vi "v5.4.vi"() -> ()   [LabVIEW 2018]
uses:
  <vilib>/DAQmx/read.llb/DAQmx Read (Analog 1D DBL NChan 1Samp).vi
  <extravilib>/ChannelInstances/Lossy Stream-c(a[.](c(dbl,dbl,dbl,dbl)),stamp,a[.](dbl),c(dbl,dbl,dbl,dbl,dbl,dbl,dbl))/Read With Abort.vi
  <extravilib>/ChannelInstances/High Speed Stream-c(a[.](c(dbl,dbl,dbl,dbl)),stamp,a[.](dbl),c(dbl,dbl,dbl,dbl,dbl,dbl,dbl))/_Read For Replicate.vi
  <extravilib>/ChannelInstances/Lossy Stream-c(a[.](c(dbl,dbl,dbl,dbl)),stamp,a[.](dbl),c(dbl,dbl,dbl,dbl,dbl,dbl,dbl))/Write With Abort.vi
  <extravilib>/ChannelInstances/Lossy Stream-c(a[.](c(dbl,dbl,dbl,dbl)),stamp,a[.](dbl),c(dbl,dbl,dbl,dbl,dbl,dbl,dbl))/EndpointRead.vi
  <extravilib>/ChannelInstances/Lossy Stream-c(a[.](c(dbl,dbl,dbl,dbl)),stamp,a[.](dbl),c(dbl,dbl,dbl,dbl,dbl,dbl,dbl))/Endpoint.vi
  <extravilib>/ChannelInstances/Lossy Stream-c(a[.](c(dbl,dbl,dbl,dbl)),stamp,a[.](dbl),c(dbl,dbl,dbl,dbl,dbl,dbl,dbl))/Instantiate.vi
  <extravilib>/ChannelInstances/Lossy Stream-c(a[.](c(dbl,dbl,dbl,dbl)),stamp,a[.](dbl),c(dbl,dbl,dbl,dbl,dbl,dbl,dbl))/)Channel.vi
  <resource>/ChannelSupport/_ChannelSupport/WaitIfNeeded.vi
  <extravilib>/ChannelInstances/High Speed Stream-c(a[.](c(dbl,dbl,dbl,dbl)),stamp,a[.](dbl),c(dbl,dbl,dbl,dbl,dbl,dbl,dbl))/Instantiate.vi
  <extravilib>/ChannelInstances/High Speed Stream-c(a[.](c(dbl,dbl,dbl,dbl)),stamp,a[.](dbl),c(dbl,dbl,dbl,dbl,dbl,dbl,dbl))/)Channel.vi
  <extravilib>/ChannelInstances/High Speed Stream-c(a[.](c(dbl,dbl,dbl,dbl)),stamp,a[.](dbl),c(dbl,dbl,dbl,dbl,dbl,dbl,dbl))/Abort Signal/Init Signal.vi
  <vilib>/Utility/file.llb/Write Delimited Spreadsheet (string).vi
  <vilib>/DAQmx/create/channels.llb/DAQmx Create Channel (AI-Temperature-Thermocouple).vi
  <vilib>/DAQmx/configure/timing.llb/DAQmx Timing (Sample Clock).vi
  <vilib>/DAQmx/miscellaneous.llb/DAQmx Fill In Error Info.vi
  <extravilib>/ChannelInstances/High Speed Stream-c(a[.](c(dbl,dbl,dbl,dbl)),stamp,a[.](dbl),c(dbl,dbl,dbl,dbl,dbl,dbl,dbl)).lvlib
  <resource>/objmgr/daqmx.rc
  <extravilib>/ChannelInstances/Lossy Stream-c(a[.](c(dbl,dbl,dbl,dbl)),stamp,a[.](dbl),c(dbl,dbl,dbl,dbl,dbl,dbl,dbl)).lvlib
panel:
  in  "Rig Temperature Tab Box":enum32{"Rig Temps Live", "Alarm Thresholds"}(tab)
  out "Rig Temperatures":T1
  in  "Rig Alarm Thresholds":T1
  out "DAQ Current Time":timestamp format="%<%X>T"
  in  "UI Refresh Rate (Hz)":u32=1 min=1 max=500 step=1
  out "Line Pressures":T2(graph)
  in  "Boondoggle":dbl(slide) scale=0.0..10.0
  out "Line Temperatures":T2(graph)
  out "Stoichiometric AFR [g/s]":dbl
  in  "stop":bool
  in  "Species List":string[][](table)=[["Custom", "9999999999"], ["Methanol", "6.47"], ["Butanol", "11.2"], ["Diesel", "14.5"], ["Gasoline", "14.7"], ["Propane", "15.67"], ["Methane", "13.19"], ["Hydrogen", "34.3"], ["Ammonia", "6.0466"], ["Pentane", "15.32"], ["Butane", "14.98"], ["Hexane", "15.24"], ["Ethanol", "9"], ["Empty (Not Used)", "0"]]
  in  "Lines Tab Control\n(Don't delete)":enum32{"Live Data", "AFR Info", "Setup Lines"}(tab)
  out "Flowrate Data":T3(array[cluster])
  out "AFR Display":T4(array[cluster])
  in  "Line Setup":T5(array[cluster])
  out "Actual Sample Rate":dbl
  out "Export Timestamp":timestamp format="%<%H:%M:%S>T"
  out "UI Timestamp":timestamp format="%<%X\n%x>T"
  in  "file path (dialog if empty)":path
  out "Export Loop Status":T6(ring)
  in  "Start Recording?":bool
  in  "Stop Recording?":bool
  out "Aquisition\nLoop Status":T7(ring)
  in  "OK Button":bool
  in  "DAQ Properties":cluster{"Sample Rate [Hz]":dbl}={"Sample Rate [Hz]"=1.0} {"Sample Rate [Hz]" min=1.0 max=500.0 step=1.0}
  # "Rig Temperatures [ °C]"
  # "Rig Alarm Thresholds [ °C]"
  # "Live \n Live Line Data"
  # "Air-to-Fuel Ratios for each Line"
  # "Line Setup"
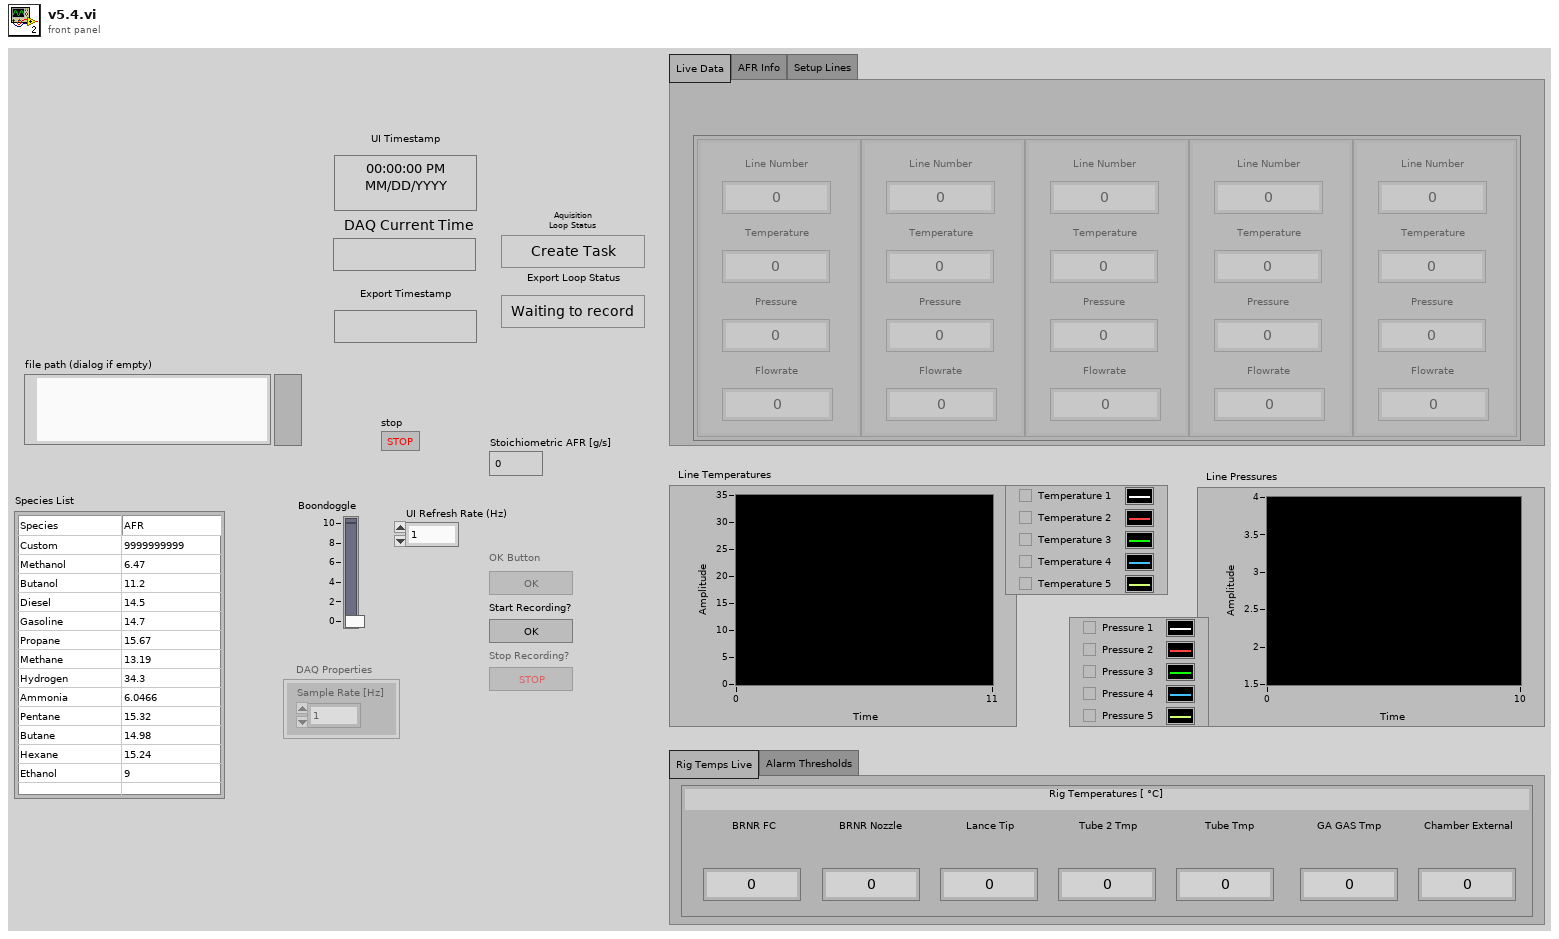
[diagram p1: front panel]
types:
  T1 = cluster{"BRNR FC":dbl, "BRNR Nozzle":dbl, "Lance Tip":dbl, "Tube 2 Tmp":dbl, "Tube Tmp":dbl, "GA GAS Tmp":dbl, "Chamber External":dbl}
  T2 = cluster{"[0]":dbl, "[1]":dbl, "[2]":dbl, "[3]":dbl, "[4]":dbl}
  T3 = cluster{"Line Number":dbl, "Temperature":dbl, "Pressure":dbl, "Flowrate":dbl}[]
  T4 = cluster{"Line Number":i32, "AFR":dbl, "Species":enum16{"Empty (Not used)", "Custom", "Methanol", "Ethanol", "Butanol", "Diesel", "Gasoline", "Propane", "Methane", "Hydrogen", "Pentane", "Butane", "Hexane"}}[]
  T5 = cluster{"Custom AFR":dbl, "Species":enum16{"Empty (Not used)", "Custom", "Methanol", "Ethanol", "Butanol", "Diesel", "Gasoline", "Propane", "Methane", "Hydrogen", "Pentane", "Butane", "Hexane"}}[]
  T6 = enum16{"Waiting to record", "Creating Spreadsheet", "Recording", "Finished Recording"}
  T7 = enum16{"Create Task", "Change Settings", "Check Settings", "Read Data", "End Task"}
  T8 = enum8{"Enabled", "Disabled", "Disabled and Grayed Out"}
  T9 = cluster{"Line":i32, "AFR":dbl, "Species":enum16{"Empty (Not used)", "Custom", "Methanol", "Ethanol", "Butanol", "Diesel", "Gasoline", "Propane", "Methane", "Hydrogen", "Pentane", "Butane", "Hexane"}}
  T10 = enum16{"Empty (Not used)", "Custom", "Methanol", "Ethanol", "Butanol", "Diesel", "Gasoline", "Propane", "Methane", "Hydrogen", "Pentane", "Butane", "Hexane"}
  T11 = cluster{"Flowrate Data":cluster{"Line Number":dbl, "Temperature":dbl, "Pressure":dbl, "Flowrate":dbl}[], "Current Time":timestamp, "DAQmx Data":dbl[], "Rig Temperatures":cluster{"BRNR FC":dbl, "BRNR Nozzle":dbl, "Lance Tip":dbl, "Tube 2 Tmp":dbl, "Tube Tmp":dbl, "GA GAS Tmp":dbl, "Chamber External Temp":dbl}}
  T12 = cluster{"BRNR FC":dbl, "BRNR Nozzle":dbl, "Lance Tip":dbl, "Tube 2 Tmp":dbl, "Tube Tmp":dbl, "GA GAS Tmp":dbl, "Chamber External Temp":dbl}
  T13 = typedef "High Speed Stream-c(a[.](c(dbl,dbl,dbl,dbl)),stamp,a[.](dbl),c(dbl,dbl,dbl,dbl,dbl,dbl,dbl)).lvlib/)Channel.ctl" = refnum<queue>
  T14 = typedef "Lossy Stream-c(a[.](c(dbl,dbl,dbl,dbl)),stamp,a[.](dbl),c(dbl,dbl,dbl,dbl,dbl,dbl,dbl)).lvlib/)Channel.ctl" = refnum<queue>
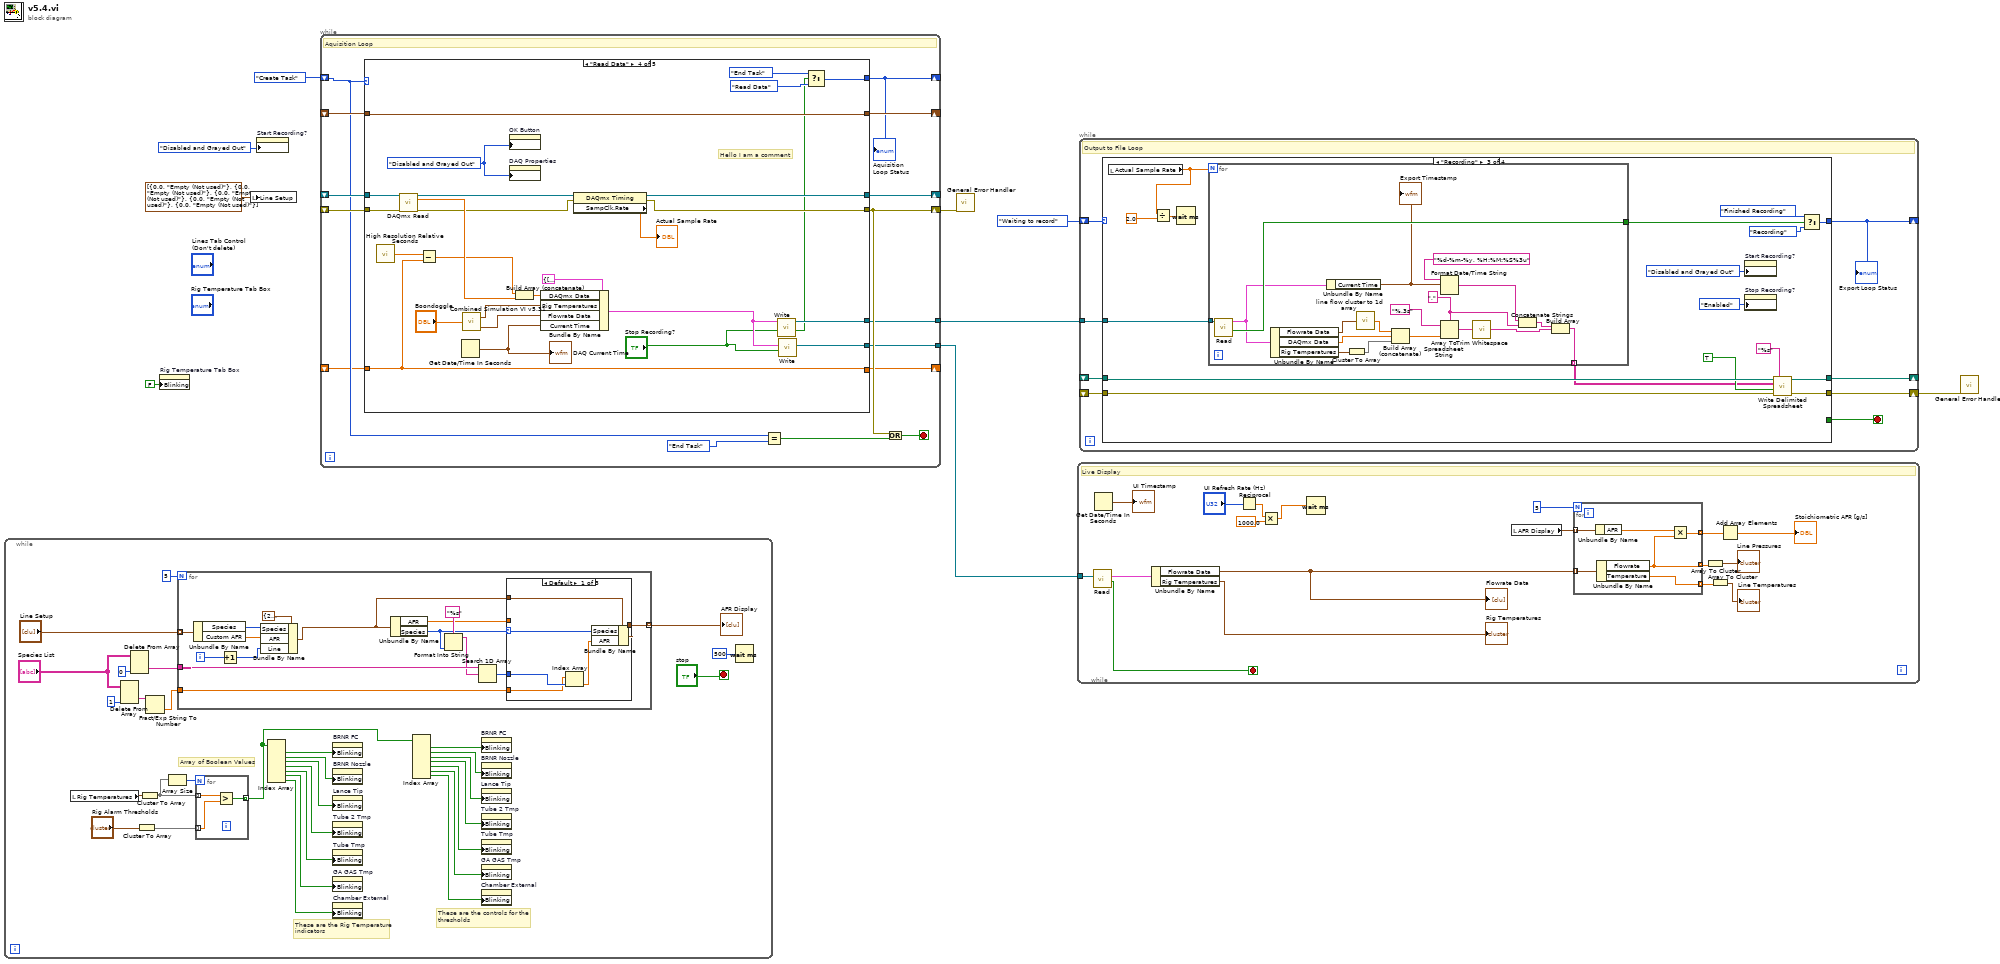
[diagram p0: block diagram]
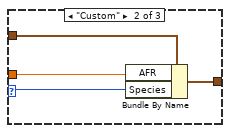
[diagram p2: hidden frame]
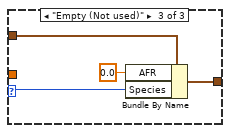
[diagram p3: hidden frame]
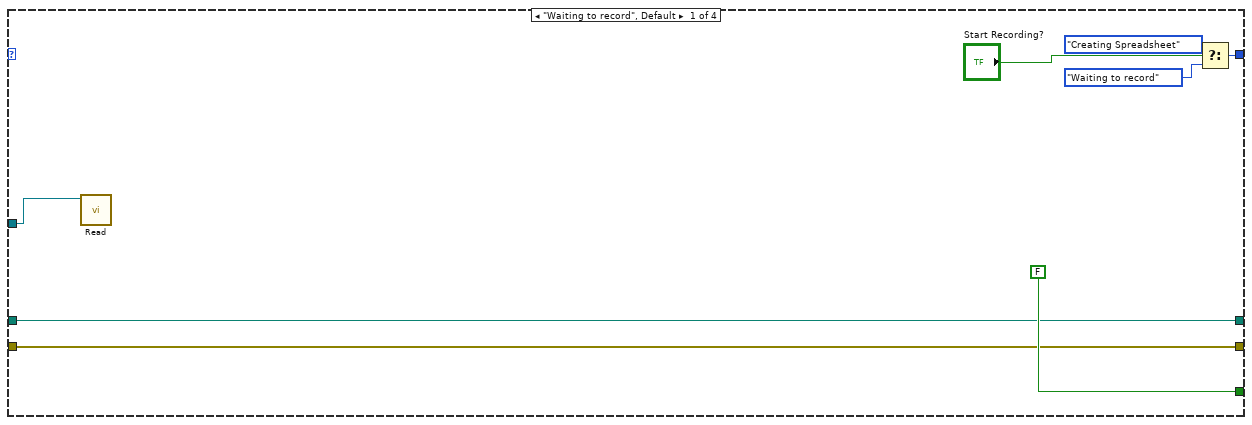
[diagram p4: hidden frame]
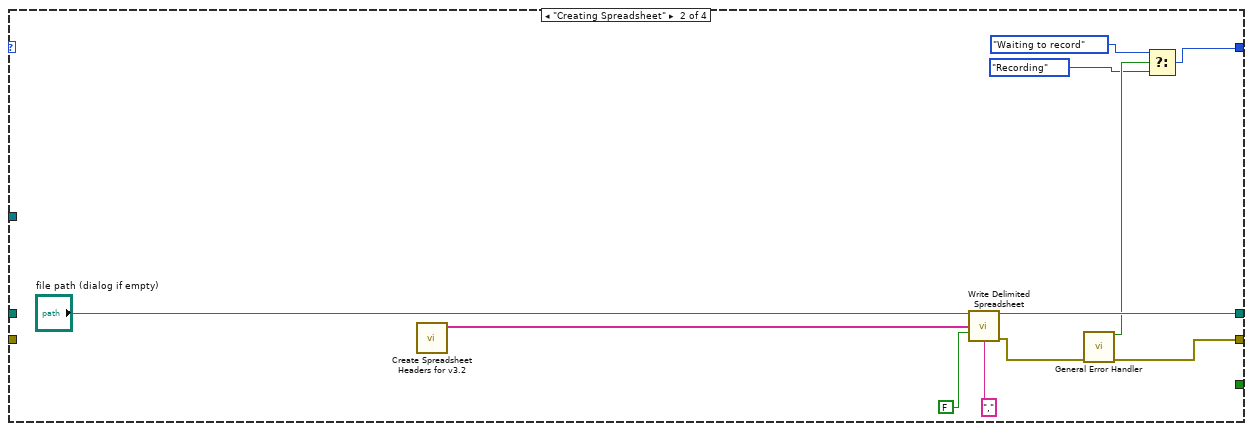
[diagram p5: hidden frame]
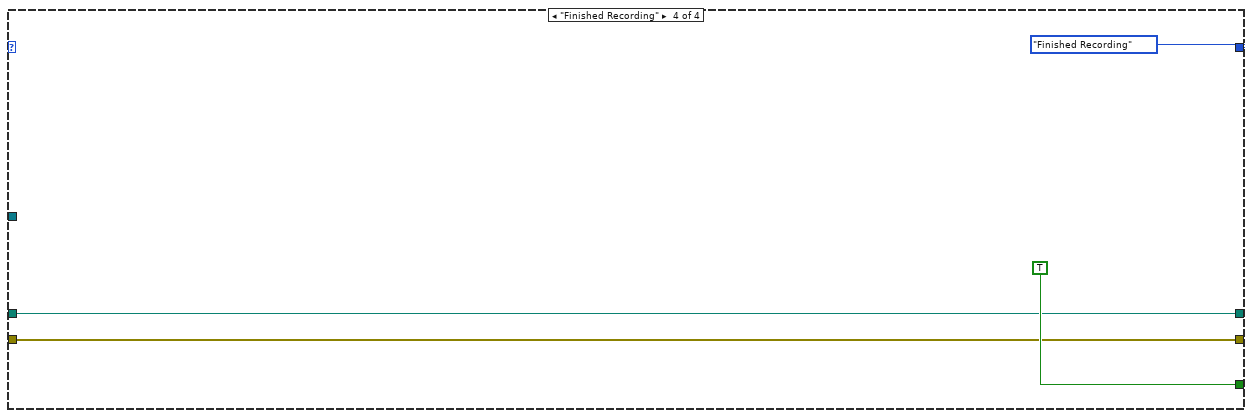
[diagram p6: hidden frame]
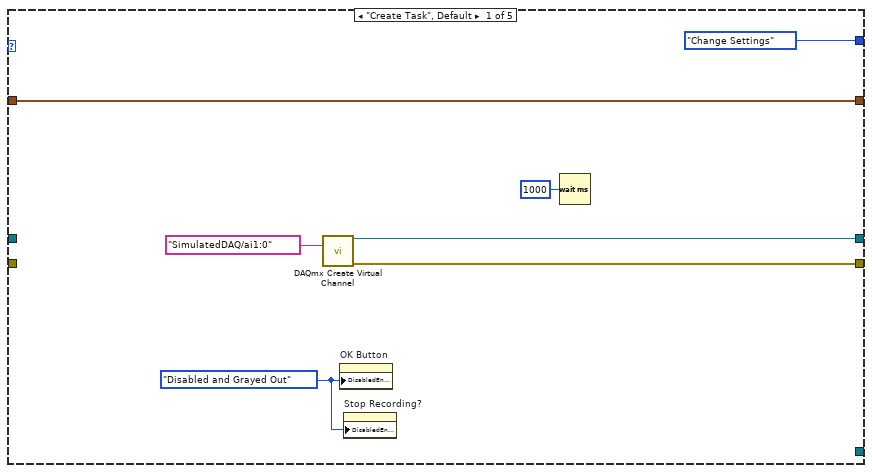
[diagram p7: hidden frame]
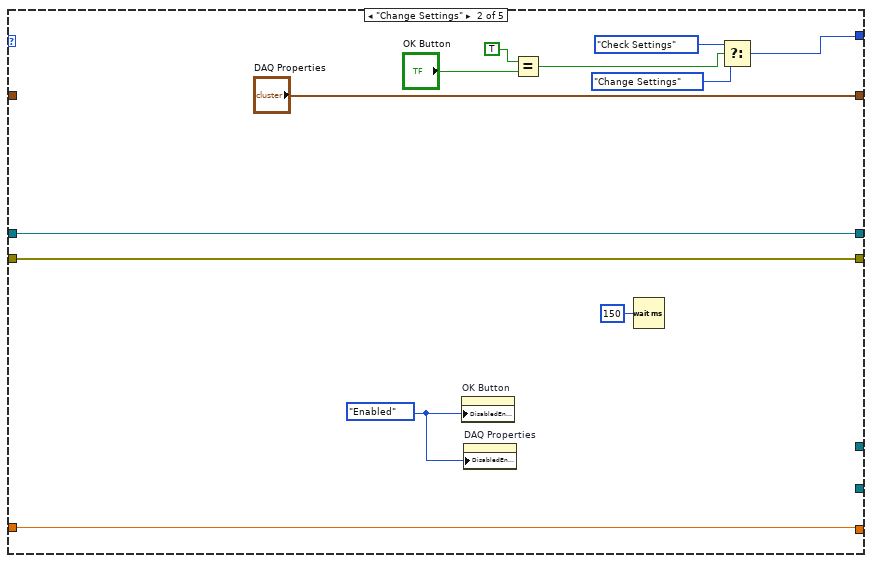
[diagram p8: hidden frame]
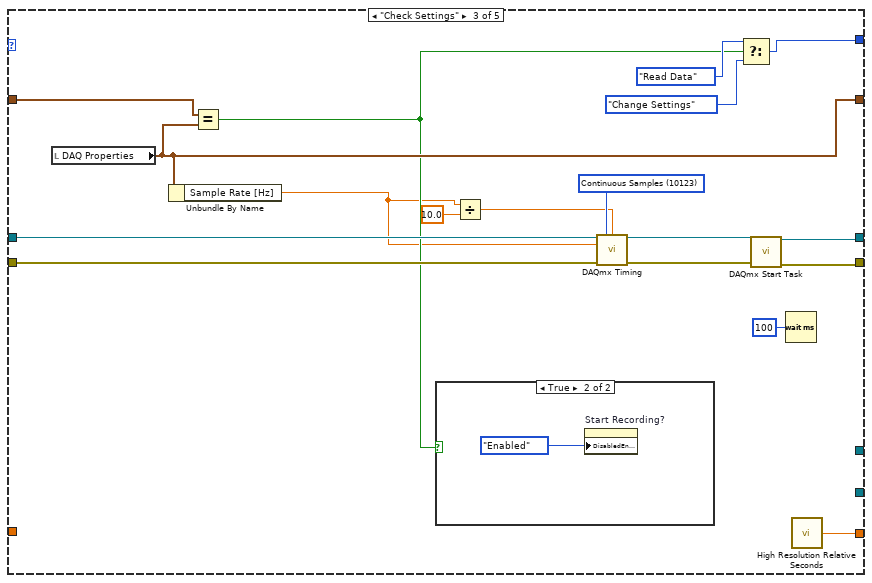
[diagram p9: hidden frame]
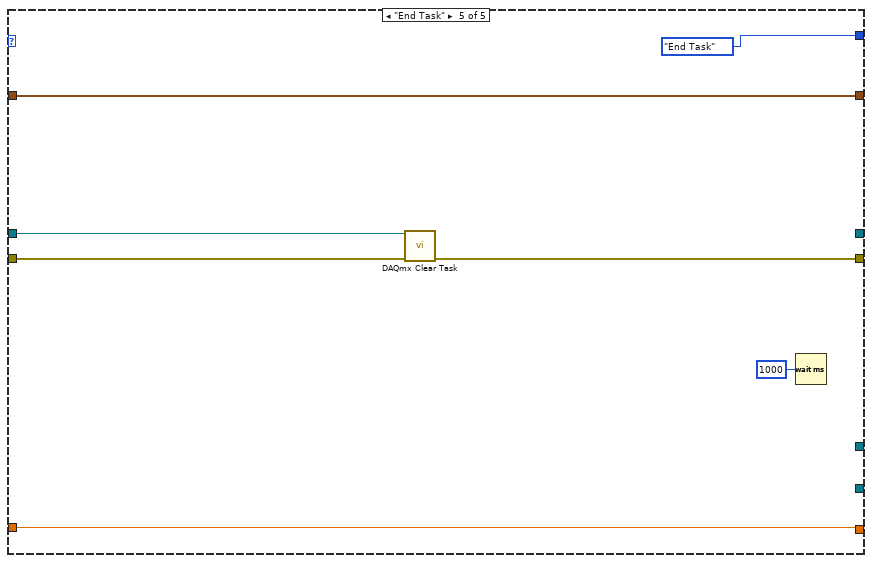
[diagram p11: hidden frame]
diagram:
  n1 = while {
    stop <- "stop" stop-if-true
    # "Array of Boolean Values"
    # "These are the controls for the \nthresholds"
    # "These are the Rig Temperature\nindicators"
    n2 = local read "Rig Temperatures"() -> (w28:T1)
    n3 = Delete From Array(array="Species List", index (col)=1 ("disabled index (col)")) -> (deleted portion=w35:string[])  [unwired: 2 in, 1 out]
    n4 = Delete From Array(array="Species List", index (col)=0) -> (deleted portion=w36:string[])  [unwired: 2 in, 1 out]
    n5 = Cluster To Array(cluster="Rig Alarm Thresholds") -> (array=w27:dbl[])
    n6 = Cluster To Array(cluster=w28) -> (array=w25:dbl[])
    n7 = Fract/Exp String To Number(string=w35) -> (number=w34:dbl[])  [unwired: 3 in, 1 out]
    n8 = Array Size(array=w25) -> (size(s)=w26:i32)
    n9 = for {
      N: 5 -> [_]
      tunnel: w36 -> [w57]
      tunnel: w34 -> [w54]
      tunnel: "Line Setup" -> [w47] mode=indexing
      tunnel: [w44] -> w30 mode=indexing
      i -> [w46]
      n10 = Unbundle By Name(w47) -> ("Species"=w51:T10, "Custom AFR"=w50:dbl)
      n11 = Increment(x=w46) -> (x+1=w48:i32)
      n12 = Bundle By Name(cluster=T9 {"Line"=2, "AFR"=1.0, "Species"=enum."Pentane"} ("AFR Inputs"), "Species"=w51, "AFR"=w50, "Line"=w48) -> (w45:T9)
      n13 = Unbundle By Name(w45) -> ("AFR"=w55:dbl, "Species"=w52:T10)
      n14 = Format Into String(format string="%s", w52) -> (resulting string=w56:string)  [unwired: 2 in, 1 out]
      n15 = Search 1D Array(1D array=w57, element=w56) -> (index of element=w53:i32)  [unwired: 1 in]
      n16 = case shown="Default" w52 {
        selector: w52 -> [w61 w65 w70]
        tunnel: w55 -> [_ w68 _]
        tunnel: w54 -> [w63 _ _]
        tunnel: w53 -> [w64 _ _]
        tunnel: [w59 w67 w72] -> w44
        tunnel: w45 -> [w60 w66 w71]
        frame Default {
          n17 = Index Array(array=w63, index=w64) -> (element=w62:dbl)
          n18 = Bundle By Name(cluster=w60, "Species"=w61, "AFR"=w62) -> (w59:T9)
        }
        frame "Custom" {
          n19 = Bundle By Name(cluster=w66, "AFR"=w68, "Species"=w65) -> (w67:T9)
        }
        frame "Empty (Not used)" {
          n20 = Bundle By Name(cluster=w71, "AFR"=0.0, "Species"=w70) -> (w72:T9)
        }
      }
    }
    "AFR Display" <- w30
    n21 = for {
      N: w26 -> [_]
      tunnel: w27 -> [w42] mode=indexing
      tunnel: w25 -> [w43] mode=indexing
      tunnel: [w41] -> w17 mode=indexing
      n22 = Greater?(x=w43, y=w42) -> (0:w41:bool)
    }
    n23 = Index Array(array=w17) -> (element #1=w24:bool, element #2=w23:bool, element #3=w22:bool, element #4=w21:bool, element #5=w20:bool, element #6=w19:bool, element #7=w18:bool)  [unwired: 7 in]
    n24 = property on="BRNR FC" class="DigNum (strict)"("Blinking"=w24) -> ()  [unwired: 2 in, 2 out]
    n25 = property on="BRNR Nozzle" class="DigNum (strict)"("Blinking"=w23) -> ()  [unwired: 2 in, 2 out]
    n26 = property on="Lance Tip" class="DigNum (strict)"("Blinking"=w22) -> ()  [unwired: 2 in, 2 out]
    n27 = property on="Tube 2 Tmp" class="DigNum (strict)"("Blinking"=w21) -> ()  [unwired: 2 in, 2 out]
    n28 = property on="Tube Tmp" class="DigNum (strict)"("Blinking"=w20) -> ()  [unwired: 2 in, 2 out]
    n29 = property on="GA GAS Tmp" class="DigNum (strict)"("Blinking"=w19) -> ()  [unwired: 2 in, 2 out]
    n30 = property on="Chamber External" class="DigNum (strict)"("Blinking"=w18) -> ()  [unwired: 2 in, 2 out]
    n31 = Index Array(array=w17) -> (element #1=w16:bool, element #2=w15:bool, element #3=w14:bool, element #4=w13:bool, element #5=w12:bool, element #6=w11:bool, element #7=w10:bool)  [unwired: 7 in]
    n32 = property on="BRNR FC" class="DigNum (strict)"("Blinking"=w16) -> ()  [unwired: 2 in, 2 out]
    n33 = property on="BRNR Nozzle" class="DigNum (strict)"("Blinking"=w15) -> ()  [unwired: 2 in, 2 out]
    n34 = property on="Lance Tip" class="DigNum (strict)"("Blinking"=w14) -> ()  [unwired: 2 in, 2 out]
    n35 = property on="Tube 2 Tmp" class="DigNum (strict)"("Blinking"=w13) -> ()  [unwired: 2 in, 2 out]
    n36 = property on="Tube Tmp" class="DigNum (strict)"("Blinking"=w12) -> ()  [unwired: 2 in, 2 out]
    n37 = property on="GA GAS Tmp" class="DigNum (strict)"("Blinking"=w11) -> ()  [unwired: 2 in, 2 out]
    n38 = property on="Chamber External" class="DigNum (strict)"("Blinking"=w10) -> ()  [unwired: 2 in, 2 out]
    n39 = Wait (ms)(milliseconds to wait=u32 500) -> ()  [unwired: 1 out]
  }
  n40 = property on="Rig Temperature Tab Box" class="TabCtl (strict)"("Blinking"=FALSE) -> ()  [unwired: 2 in, 2 out]
  n41 = local write "Line Setup"(T5 [{"Custom AFR"=0.0, "Species"=enum."Empty (Not used)"}, {"Custom AFR"=0.0, "Species"=enum."Empty (Not used)"}, {"Custom AFR"=0.0, "Species"=enum."Empty (Not used)"}, {"Custom AFR"=0.0, "Species"=enum."Empty (Not used)"}, {"Custom AFR"=0.0, "Species"=enum."Empty (Not used)"}] ("Line Setup 2")) -> ()
  n42 = property on="Start Recording?" class="Bool"("DisabledEnum"=T8."Disabled and Grayed Out" ("Disabled")) -> ()  [unwired: 2 in, 2 out]
  n43 = while {
    shift-right: [w82] -> _
    shift-left: T7."Create Task" -> [w78]
    shift-right: [w87] -> _
    shift-left: _ -> [w85]
    shift-right: [w81] -> w5
    shift-left: _ -> [w84]
    shift-right: [w86] -> _
    shift-left: _ -> [w83]
    tunnel: [w77] -> w7
    tunnel: [w75] -> w3
    shift-right: [w73] -> _
    shift-left: _ -> [w74]
    stop <- w76 stop-if-true
    # "Aquisition Loop"
    n44 = case shown="\"Read Data\"" w78 {
      tunnel: [w94 w106 w114 w139 _] -> w87
      tunnel: [w93 w105 w113 w140 w159] -> w81
      tunnel: [T7."Change Settings" w99 w120 w148 T7."End Task"] -> w82
      tunnel: [w90 "DAQ Properties" w117 w150 w158] -> w86
      tunnel: w85 -> [_ w106 w119 w152 w156]
      tunnel: w84 -> [_ w105 w118 w151 w155]
      tunnel: w83 -> [w90 _ w124 w150 w158]
      tunnel: [_ _ _ w144 _] -> w77
      tunnel: [_ w95 w107 w135 w153] -> w73
      tunnel: w74 -> [_ w95 _ w135 w153]
      tunnel: [_ _ _ w132 _] -> w75
      frame "Create Task", Default {
        w88 = T8."Disabled and Grayed Out" ("Disabled")
        n45 = call-poly <vilib>:"DAQmx Create Virtual Channel.vi"("physical channels"=tag "SimulatedDAQ/ai1:0") -> ("task out"=w94:refnum<k21>, "error out"=w93:errorcluster)  [unwired: 13 in]
        n46 = property on="OK Button" class="Bool"("DisabledEnum"=w88) -> ()  [unwired: 2 in, 2 out]
        n47 = property on="Stop Recording?" class="Bool"("DisabledEnum"=w88) -> ()  [unwired: 2 in, 2 out]
        n48 = Wait (ms)(milliseconds to wait=u32 1000) -> ()  [unwired: 1 out]
      }
      frame "Change Settings" {
        w96 = T8."Enabled" ("Disabled")
        n49 = property on="OK Button" class="Bool"("DisabledEnum"=w96) -> ()  [unwired: 2 in, 2 out]
        n50 = property on="DAQ Properties" class="Clust (strict)"("DisabledEnum"=w96) -> ()  [unwired: 2 in, 2 out]
        n51 = Equal?(x=TRUE, y="OK Button") -> (x = y?=w101:bool)
        n52 = Wait (ms)(milliseconds to wait=u32 150) -> ()  [unwired: 1 out]
        n53 = Select(t=T7."Check Settings", s=w101, f=T7."Change Settings") -> (s? t:f=w99:T7)
      }
      frame "Check Settings" {
        w112 = 10123 items=["Finite Samples"=10178, "Continuous Samples"=10123, "Hardware Timed Single Point"=12522] ("sample mode")
        n54 = local read "DAQ Properties"() -> (w117:cluster{"Sample Rate [Hz]":dbl})
        n55 = Unbundle By Name(w117) -> ("Sample Rate [Hz]"=w109:dbl)
        n56 = Equal?(x=w124, y=w117) -> (x = y?=w111:bool)
        n57 = case shown="True" w111 {
          frame False {
          }
          frame True {
            n58 = property on="Start Recording?" class="Bool"("DisabledEnum"=T8."Enabled" ("Disabled")) -> ()  [unwired: 2 in, 2 out]
          }
        }
        n59 = Divide(x=w109, y=10.0) -> (x/y=w108:dbl)
        n60 = call-poly <vilib>:"DAQmx Timing.vi"("task/channels in"=w119, "sample mode"=w112, "samples per channel"=w108, "rate"=w109, "error in"=w118) -> ("task out"=w116:refnum<k21>, "error out"=w115:errorcluster)  [unwired: 9 in]
        n61 = Select(t=T7."Read Data", s=w111, f=T7."Change Settings") -> (s? t:f=w120:T7)
        n62 = call <vilib>:"DAQmx Start Task.vi"("task/channels in"=w116, "error in"=w115) -> ("task out"=w114:refnum<k21>, "error out"=w113:errorcluster)  [unwired: 12 in]
        n63 = Wait (ms)(milliseconds to wait=u32 100) -> ()  [unwired: 1 out]
        n64 = call <vilib>:"High Resolution Relative Seconds.vi"() -> ("relative seconds"=w107:dbl)
      }
      frame "Read Data" {
        w143 = T8."Disabled and Grayed Out" ("Disabled")
        # "Hello I am a comment"
        n65 = call <vilib>:"High Resolution Relative Seconds.vi"() -> ("relative seconds"=w137:dbl)
        n66 = call-poly <vilib>:"DAQmx Read.vi"("task/channels in"=w152, "error in"=w151) -> ("task out"=w141:refnum<k21>, "data"=w146:dbl[], "error out"=w138:errorcluster)  [unwired: 11 in]
        n67 = Subtract(x=w137, y=w135) -> (x-y=w136:dbl)
        n68 = Get Date/Time In Seconds() -> (seconds since 1Jan1904=w127:timestamp)
        "DAQ Current Time" <- w127
        n69 = call "Combined Simulation VI v5.31.vi"("Boondoggle Input"="Boondoggle") -> ("Rig Temperatures Cluster"=w126:T12, "Line Data (Array of Clusters)"=w128:T3)
        n70 = property on="OK Button" class="Bool"("DisabledEnum"=w143) -> ()  [unwired: 2 in, 2 out]
        n71 = property on="DAQ Properties" class="Clust (strict)"("DisabledEnum"=w143) -> ()  [unwired: 2 in, 2 out]
        n72 = Build Array (concatenate)(w136, w146) -> (w130:dbl[])
        n73 = Bundle By Name(cluster=T11 {"Flowrate Data"=[{"Line Number"=1.0, "Temperature"=17.480721541683437, "Pressure"=24.0, "Flowrate"=0.0}, {"Line Number"=2.0, "Temperature"=21.850901927104296, "Pressure"=30.0, "Flowrate"=0.0}, {"Line Number"=3.0, "Temperature"=26.221082312525155, "Pressure"=36.0, "Flowrate"=0.0}, {"Line Number"=4.0, "Temperature"=30.591262697946018, "Pressure"=42.00000000000001, "Flowrate"=0.0}, {"Line Number"=5.0, "Temperature"=34.96144308336687, "Pressure"=48.0, "Flowrate"=0.0}], "Current Time"=timestamp(0 s since 1904-01-01), "DAQmx Data"=[], "Rig Temperatures"={"BRNR FC"=0.0, "BRNR Nozzle"=0.0, "Lance Tip"=0.0, "Tube 2 Tmp"=0.0, "Tube Tmp"=0.0, "GA GAS Tmp"=0.0, "Chamber External Temp"=0.0}}, "DAQmx Data"=w130, "Rig Temperatures"=w126, "Flowrate Data"=w128, "Current Time"=w127) -> (w142:T11)
        n74 = property class="DAQmx Timing"(reference=w141, error in=w138) -> (reference out=w139:refnum<k21>, error out=w140:errorcluster, "SampClk.Rate"=→"Actual Sample Rate":dbl)
        n75 = call <extravilib>:"Write.vi"("last element? (F)"="Stop Recording?", "element"=w142) -> ("done?"=w131:bool, "channel"=w144:T13)  [unwired: 7 in, 1 out]
        n76 = call <extravilib>:"Write.vi"("last element? (F)"="Stop Recording?", "element"=w142) -> ("channel"=w132:T14)  [unwired: 7 in, 2 out]
        n77 = Select(t=T7."End Task", s=w131, f=T7."Read Data") -> (s? t:f=w148:T7)
      }
      frame "End Task" {
        n78 = call <vilib>:"DAQmx Clear Task.vi"("task in"=w156, "error in"=w155) -> ("error out"=w159:errorcluster)  [unwired: 13 in]
        n79 = Wait (ms)(milliseconds to wait=u32 1000) -> ()  [unwired: 1 out]
      }
    }
    "Aquisition\nLoop Status" <- w82
    n80 = Equal?(x=w78, y=T7."End Task") -> (x = y?=w79:bool)
    n81 = Or(x=w81, y=w79) -> (x .or. y?=w76:bool)
  }
  n82 = call <vilib>:"General Error Handler.vi"("error in (no error)"=w5) -> ()  [unwired: 10 in, 5 out]
  n83 = while {
    tunnel: w3 -> [w168]
    stop <- w164 stop-if-true
    # "Live Display"
    n84 = call <extravilib>:"Read.vi"("channel"=w168) -> ("last element?"=w164:bool, "element"=w167:T11)  [unwired: 5 in, 4 out]
    n85 = Get Date/Time In Seconds() -> (seconds since 1Jan1904=→"UI Timestamp":timestamp)
    n86 = Unbundle By Name(w167) -> ("Flowrate Data"=w165:T3, "Rig Temperatures"=→"Rig Temperatures":T12)
    "Flowrate Data" <- w165
    n87 = Reciprocal(x="UI Refresh Rate (Hz)") -> (1/x=w161:dbl)
    n88 = Multiply(x=w161, y=1000.0) -> (x*y=w160:dbl)
    n89 = Wait (ms)(milliseconds to wait=w160) -> ()  [unwired: 1 out]
    n90 = local read "AFR Display"() -> (w175:T4)
    n91 = for {
      N: 5 -> [_]
      tunnel: w175 -> [w183] mode=indexing
      tunnel: [w181] -> w174 mode=indexing
      tunnel: [w180] -> w171 mode=indexing
      tunnel: [w179] -> w172 mode=indexing
      tunnel: w165 -> [w178] mode=indexing
      n92 = Unbundle By Name(w183) -> ("AFR"=w182:dbl)
      n93 = Unbundle By Name(w178) -> ("Flowrate"=w179:dbl, "Temperature"=w180:dbl)
      n94 = Multiply(x=w182, y=w179) -> (x*y=w181:dbl)
    }
    n95 = Array To Cluster(array=w172) -> (cluster=→"Line Pressures":T2)
    n96 = Array To Cluster(array=w171) -> (cluster=→"Line Temperatures":T2)
    n97 = Add Array Elements(numeric array=w174) -> (sum=→"Stoichiometric AFR [g/s]":dbl)
  }
  n98 = while {
    shift-right: [w191] -> _
    shift-left: T6."Waiting to record" -> [w190]
    tunnel: w7 -> [w188]
    shift-right: [w186] -> _
    shift-left: _ -> [w187]
    shift-right: [w185] -> w6
    shift-left: _ -> [w184]
    stop <- w189 stop-if-true
    # "Output to File Loop"
    n99 = case shown="\"Recording\"" w190 {
      tunnel: [w196 w202 w226 T6."Finished Recording"] -> w191
      tunnel: [FALSE _ _ TRUE] -> w189
      tunnel: w188 -> [w192 _ w223 _]
      tunnel: w187 -> [w194 _ w220 w247]
      tunnel: [w194 w210 w221 w247] -> w186
      tunnel: [w193 w204 w216 w246] -> w185
      tunnel: w184 -> [w193 _ w219 w246]
      frame "Waiting to record", Default {
        n100 = call <extravilib>:"Read.vi"("channel"=w192) -> ()  [unwired: 6 in, 5 out]
        n101 = Select(t=T6."Creating Spreadsheet", s="Start Recording?", f=T6."Waiting to record") -> (s? t:f=w196:T6)
      }
      frame "Creating Spreadsheet" {
        n102 = call "Create Spreadsheet Headers for v3.2.vi"() -> ("Array"=w209:string[])  [unwired: 11 in]
        n103 = call-poly <vilib>:"Write Delimited Spreadsheet.vi"("file path (dialog if empty)"="file path (dialog if empty)", "1D data"=w209, "append to file? (new file:F)"=FALSE, "delimiter (\\t)"="," ("delimiter (\\t)")) -> ("new file path (Not A Path if cancelled)"=w210:path, "error out"=w205:errorcluster)  [unwired: 10 in]
        n104 = call <vilib>:"General Error Handler.vi"("error in (no error)"=w205) -> ("error?"=w203:bool, "error out"=w204:errorcluster)  [unwired: 10 in, 3 out]
        n105 = Select(t=T6."Waiting to record", s=w203, f=T6."Recording") -> (s? t:f=w202:T6)
      }
      frame "Recording" {
        n106 = local read "Actual Sample Rate"() -> (w212:dbl)
        n107 = Divide(x=w212, y=2.0) -> (x/y=w211:dbl)
        n108 = Wait (ms)(milliseconds to wait=w211) -> ()  [unwired: 1 out]
        n109 = for {
          N: w212 -> [_]
          tunnel: w223 -> [w244]
          tunnel: [w243] -> w222
          tunnel: [w228] -> w214 mode=indexing
          w233 = "," ("delimiter (Tab)")
          n110 = call <extravilib>:"Read.vi"("channel"=w244) -> ("done?"=w243:bool, "element"=w241:T11)  [unwired: 6 in, 3 out]
          n111 = Unbundle By Name(w241) -> ("Flowrate Data"=w242:T3, "DAQmx Data"=w239:dbl[], "Rig Temperatures"=w245:T12)
          n112 = Unbundle By Name(w241) -> ("Current Time"=w234:timestamp)
          "Export Timestamp" <- w234
          n113 = Cluster To Array(cluster=w245) -> (array=w240:dbl[])
          n114 = call "line flow cluster to 1d array.vi"("Flowrate Data"=w242) -> ("Array"=w238:dbl[])
          n115 = Build Array (concatenate)(w238, w239, w240) -> (w231:dbl[])
          n116 = Format Date/Time String(time format string (%c)="%d-%m-%y, %H:%M:%S%3u", seconds (now)=w234) -> (date/time string=w232:string)  [unwired: 1 in]
          n117 = Array To Spreadsheet String(delimiter (Tab)=w233, array=w231, 3:"%.3s" ("format string")) -> (spreadsheet string=w237:string)
          n118 = call <vilib>:"Trim Whitespace.vi"("string"=w237) -> ("trimmed string"=w229:string)  [unwired: 1 in]
          n119 = Concatenate Strings(w232, w233) -> (w230:string)
          n120 = Build Array(w230, w229) -> (w228:string[])
        }
        n121 = property on="Start Recording?" class="Bool"("DisabledEnum"=T8."Disabled and Grayed Out" ("Disabled")) -> ()  [unwired: 2 in, 2 out]
        n122 = property on="Stop Recording?" class="Bool"("DisabledEnum"=T8."Enabled" ("Disabled")) -> ()  [unwired: 2 in, 2 out]
        n123 = call-poly <vilib>:"Write Delimited Spreadsheet.vi"("file path (dialog if empty)"=w220, "format (%s)"="%s", "2D data"=w214, "append to file? (new file:F)"=TRUE, "error in (no error)"=w219) -> ("new file path (Not A Path if cancelled)"=w221:path, "error out"=w216:errorcluster)  [unwired: 9 in]
        n124 = Select(t=T6."Finished Recording", s=w222, f=T6."Recording") -> (s? t:f=w226:T6)
      }
      frame "Finished Recording" {
      }
    }
    "Export Loop Status" <- w191
  }
  n125 = call <vilib>:"General Error Handler.vi"("error in (no error)"=w6) -> ()  [unwired: 10 in, 5 out]
